vi "Initialize.vi"(8 "Error In":errorcluster, 11 "SerialComm in":refnum<class "SerialComm.lvclass">) -> (0 "Error Out":errorcluster, 3 "SerialComm out":refnum<class "SerialComm.lvclass">)   [LabVIEW 2016, in "SerialComm.lvclass"]
uses:
  SerialComm.lvclass
  <vilib>/Instr/_visa.llb/VISA Configure Serial Port (Instr).vi
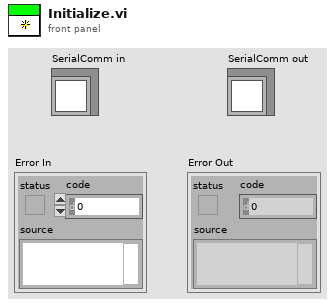
[diagram p1: front panel]
types:
  T1 = typedef "Serial - Settings.ctl" = cluster{"baud rate":u32, "data bits":u16, "parity":enum16{"None", "Odd", "Even", "Mark", "Space"}, "stop bits":u16, "flow control":u16}
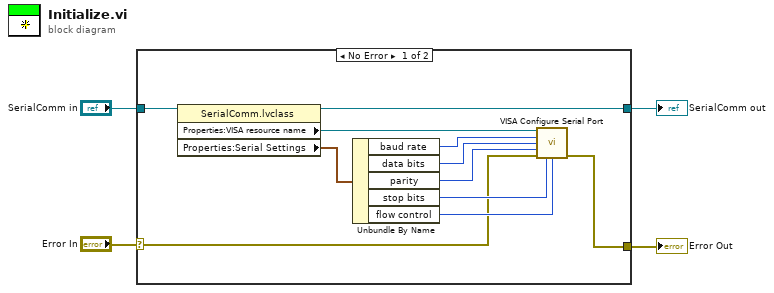
[diagram p0: block diagram]
diagram:
  n1 = case shown="No Error" "Error In" {
    selector: "Error In" -> [w6 w17]
    tunnel: [w5 w17] -> w3
    tunnel: [w14 w16] -> w1
    tunnel: "SerialComm in" -> [w15 w16]
    frame No Error {
      n2 = property class="SerialComm.lvclass"(reference=w15) -> (reference out=w14:refnum<class "SerialComm.lvclass">, "Properties:VISA resource name"=w13:refnum<visa-resource-name>, "Properties:Serial Settings"=w12:T1)  [unwired: 1 in, 1 out]
      n3 = Unbundle By Name(w12) -> ("baud rate"=w11:u32, "data bits"=w10:u16, "parity"=w9:enum16{"None", "Odd", "Even", "Mark", "Space"}, "stop bits"=w8:u16, "flow control"=w7:u16)
      n4 = call-poly "VISA Configure Serial Port"("VISA resource name"=w13, "baud rate (9600)"=w11, "data bits (8)"=w10, "parity (0:none)"=w9, "error in (no error)"=w6, "stop bits (10: 1 bit)"=w8, "flow control (0:none)"=w7) -> ("error out"=w5:errorcluster)  [unwired: 2 in, 6 out]
    }
    frame Error {
    }
  }
  "Error Out" <- w3
  "SerialComm out" <- w1
